vi "ConvertGoop1ToGoop3_KeepViPrefix.vi"(1 "OrgViName":path=path "C:/UML/GOOP2/AbstractNode_class/AbstractNode addChild.vi", 2 "ClassFolder":path=path "C:/UML/GOOP2/AbstractNode_class", 5 "error in (no error)":errorcluster, 6 "ClassPrefix":string="AbstractNode ") -> (12 "ClassFolderOut":path, 14 "Don'tUseVI":bool, 15 "KeepPrefix":bool, 16 "NewClassPath":path, 18 "NewClassPathWithPreFix":path, 19 "error out":errorcluster)   [LabVIEW 2020]
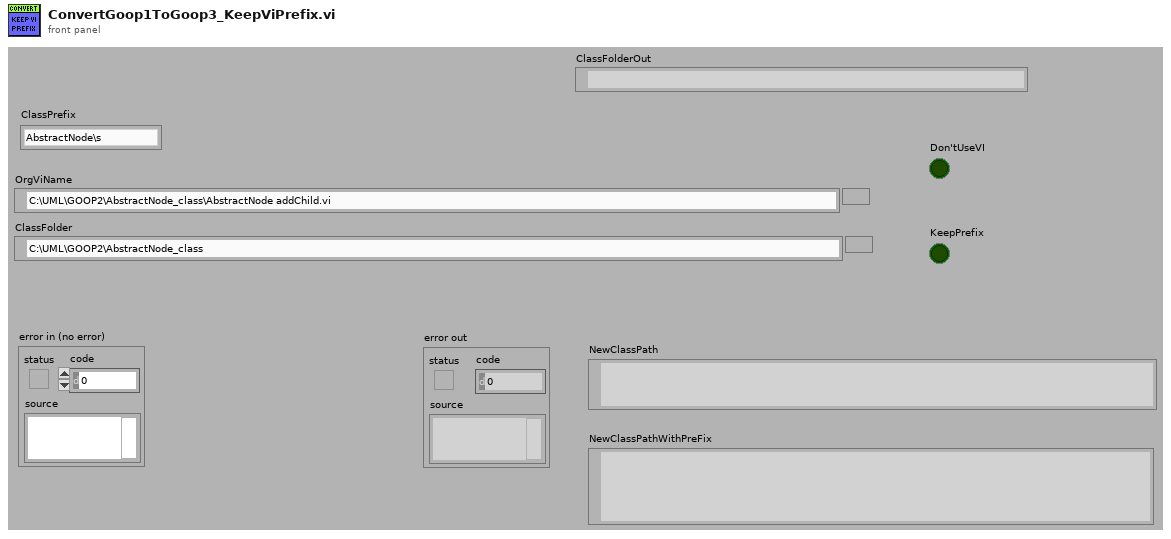
[diagram p1: front panel]
types:
  T1 = typedef "Librarian File Info Out.ctl" = cluster{"creation date":u32, "last mod date":u32, "type":string, "creator":string, "LV version":i32, "size":i32, "top level":bool}
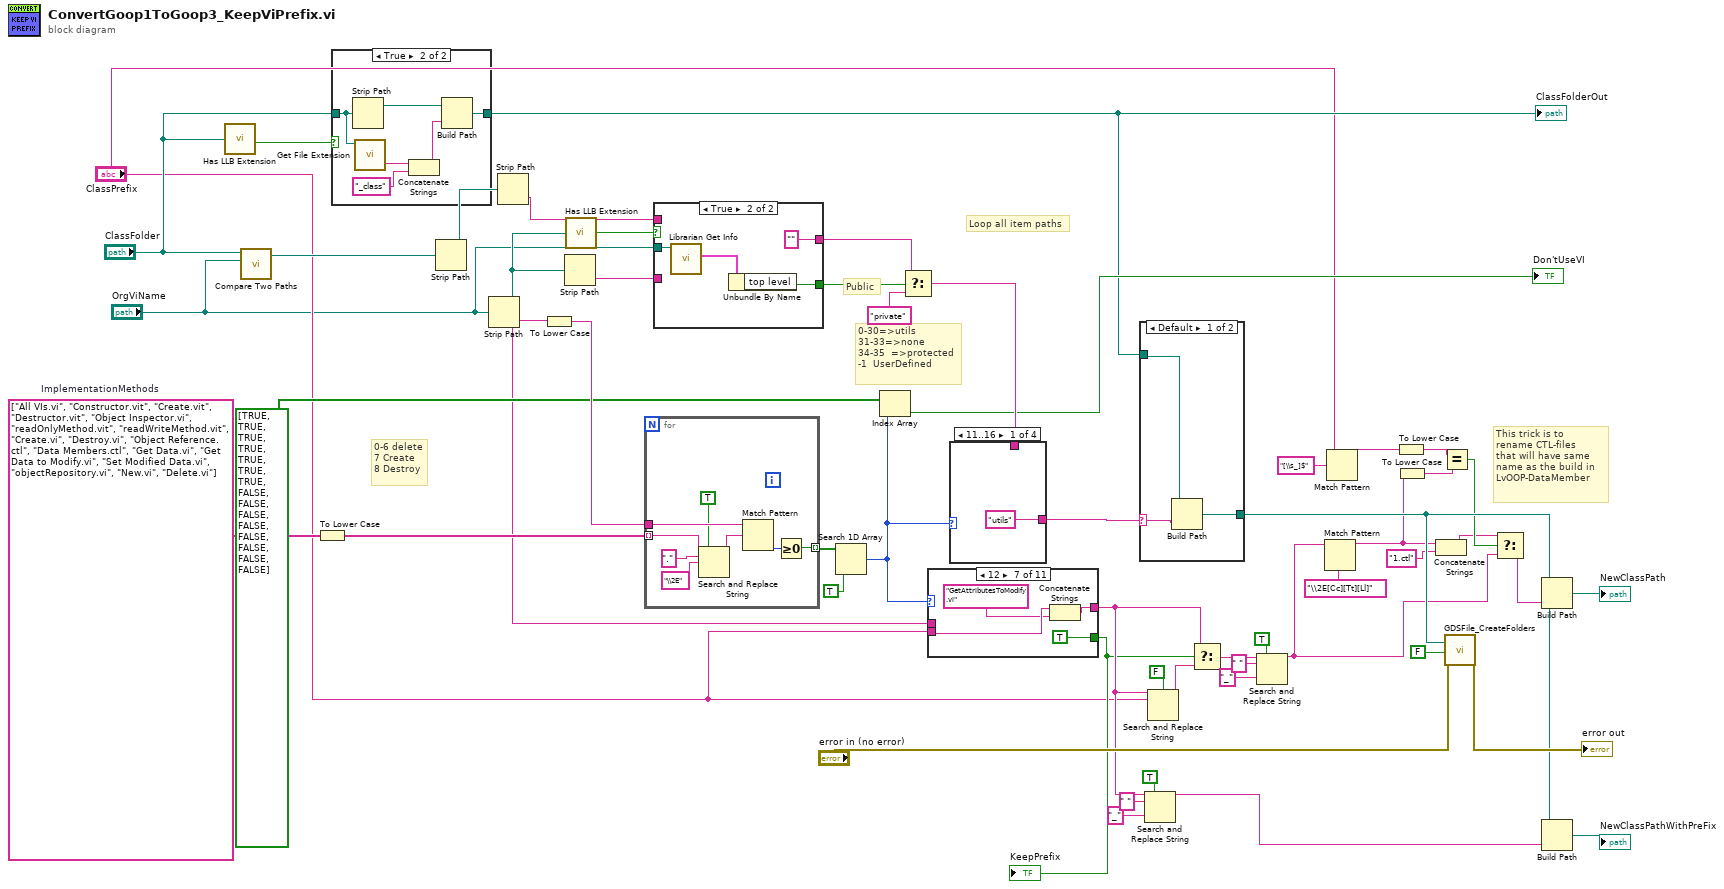
[diagram p0: block diagram]
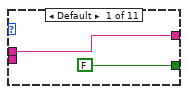
[diagram p2: hidden frame]
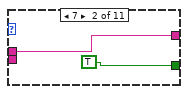
[diagram p3: hidden frame]
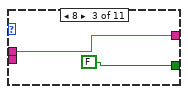
[diagram p4: hidden frame]
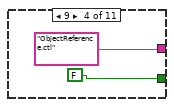
[diagram p5: hidden frame]
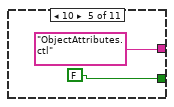
[diagram p6: hidden frame]
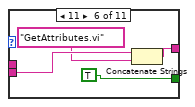
[diagram p7: hidden frame]
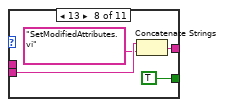
[diagram p8: hidden frame]
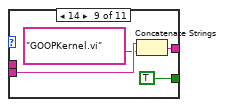
[diagram p9: hidden frame]
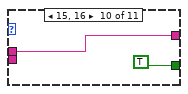
[diagram p10: hidden frame]
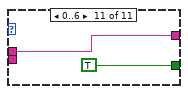
[diagram p11: hidden frame]
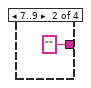
[diagram p14: hidden frame]
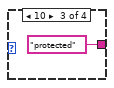
[diagram p15: hidden frame]
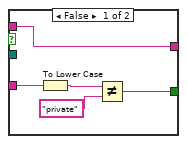
[diagram p17: hidden frame]
diagram:
  w53 = string[] ["All VIs.vi", "Constructor.vit", "Create.vit", "Destructor.vit", "Object Inspector.vi", "readOnlyMethod.vit", "readWriteMethod.vit", "Create.vi", "Destroy.vi", "Object Reference.ctl", "Data Members.ctl", "Get Data.vi", "Get Data to Modify.vi", "Set Modified Data.vi", "objectRepository.vi", "New.vi", "Delete.vi"]  # ImplementationMethods
  # "0-6 delete\n7 Create\n8 Destroy"
  # "This trick is to\nrename CTL-files\nthat will have same\nname as the build in\nLvOOP-DataMember"
  # "Public"
  # "0-30=>utils\n31-33=>none\n34-35  =>protected\n-1  UserDefined"
  # "Loop all item paths"
  n1 = call <vilib>:"Has LLB Extension.vi"("path"="ClassFolder") -> ("path to VI library?"=w20:bool)
  n2 = call <vilib>:"Compare Two Paths.vi"("Path 2"="OrgViName", "Path 1"="ClassFolder") -> ("Relative Path from 1 to 2"=w25:path)  [unwired: 6 in, 3 out]
  n3 = To Lower Case(string=w53) -> (all lower case string=w54:string[])
  n4 = case shown="True" w20 {
    tunnel: "ClassFolder" -> [w55 w61]
    tunnel: [w55 w60] -> w18
    frame False {
    }
    frame True {
      n5 = Strip Path(path=w61) -> (stripped path=w57:path)  [unwired: 1 out]
      n6 = call <vilib>:"Get File Extension.vi"("file"=w61) -> ("filename without extension"=w59:string)  [unwired: 6 in, 4 out]
      n7 = Concatenate Strings(w59, "_class" ("string")) -> (w56:string)
      n8 = Build Path(base path=w57, name or relative path=w56) -> (appended path=w60:path)
    }
  }
  "ClassFolderOut" <- w18
  n9 = Strip Path(path=w25) -> (stripped path=w24:path)  [unwired: 1 out]
  n10 = Strip Path(path="OrgViName") -> (stripped path=w50:path, name=w5:string)
  n11 = Strip Path(path=w24) -> (name=w23:string)  [unwired: 1 out]
  n12 = To Lower Case(string=w5) -> (all lower case string=w52:string)
  n13 = Strip Path(path=w50) -> (name=w47:string)  [unwired: 1 out]
  n14 = call <vilib>:"Has LLB Extension.vi"("path"=w50) -> ("path to VI library?"=w51:bool)
  n15 = for {
    tunnel: w54 -> [w68] mode=indexing
    tunnel: w52 -> [w69]
    tunnel: [w62] -> w38 mode=indexing
    n16 = Search and Replace String(replace all?=TRUE ("replace all? (F)"), input string=w68, search string=".", replace string="\\2E" ("replace string (\"\")")) -> (result string=w67:string)  [unwired: 4 in, 3 out]
    n17 = Match Pattern(string=w69, regular expression=w67) -> (offset past match=w63:i32)  [unwired: 1 in, 3 out]
    n18 = Greater Or Equal To 0?(x=w63) -> (x >= 0?=w62:bool)
  }
  n19 = case shown="True" w51 {
    tunnel: "OrgViName" -> [_ w78]
    tunnel: w47 -> [w70 _]
    tunnel: [w72 w76] -> w46
    tunnel: [w71 "" ("y")] -> w26
    tunnel: w23 -> [w71 _]
    frame False {
      n20 = To Lower Case(string=w70) -> (all lower case string=w74:string)
      n21 = Not Equal?(x=w74, y="private") -> (x != y?=w72:bool)
    }
    frame True {
      n22 = call <vilib>:"Librarian Get Info.vi"("path"=w78) -> ("file information"=w77:T1)  [unwired: 8 in, 2 out]
      n23 = Unbundle By Name(w77) -> ("top level"=w76:bool)
    }
  }
  n24 = Search 1D Array(1D array=w38, element=TRUE) -> (index of element=w6:i32)  [unwired: 1 in]
  n25 = Index Array(array=bool[] [TRUE, TRUE, TRUE, TRUE, TRUE, TRUE, TRUE, FALSE, FALSE, FALSE, FALSE, FALSE, FALSE, FALSE, FALSE] (".not. x?"), index=w6) -> (element=→"Don'tUseVI":bool)
  n26 = Select(t=w26, s=w46, f="private" ("y")) -> (s? t:f=w44:string)
  n27 = case shown="12" w6 {
    tunnel: w5 -> [w80 w82 w84 _ _ _ _ _ _ w106 w108]
    tunnel: [w80 w82 w84 "ObjectReference.ctl" ("name") "ObjectAttributes.ctl" ("name") w89 w93 w97 w101 w106 w108] -> w4
    tunnel: [FALSE ("replace all? (F)") TRUE ("ignore case? (F)") FALSE ("ignore case? (F)") FALSE ("ignore case? (F)") FALSE ("ignore case? (F)") TRUE ("ignore case? (F)") TRUE ("ignore case? (F)") TRUE ("ignore case? (F)") TRUE ("ignore case? (F)") TRUE ("ignore case? (F)") TRUE ("replace all? (F)")] -> w3
    tunnel: "ClassPrefix" -> [_ _ _ _ _ w91 w95 w99 w103 _ _]
    frame Default {
    }
    frame 7 {
    }
    frame 8 {
    }
    frame 9 {
    }
    frame 10 {
    }
    frame 11 {
      n28 = Concatenate Strings(w91, "GetAttributes.vi" ("name")) -> (w89:string)
    }
    frame 12 {
      n29 = Concatenate Strings(w95, "GetAttributesToModify.vi" ("name")) -> (w93:string)
    }
    frame 13 {
      n30 = Concatenate Strings(w99, "SetModifiedAttributes.vi" ("name")) -> (w97:string)
    }
    frame 14 {
      n31 = Concatenate Strings(w103, "GOOPKernel.vi" ("name")) -> (w101:string)
    }
    frame 15, 16 {
    }
    frame 0..6 {
    }
  }
  "KeepPrefix" <- w3
  n32 = case shown="11..16" w6 {
    tunnel: ["utils" "" "protected" w112] -> w43
    tunnel: w44 -> [_ _ _ w112]
    frame 11..16 {
    }
    frame 7..9 {
    }
    frame 10 {
    }
    frame Default {
    }
  }
  n33 = case shown="Default" w43 {
    selector: w43 -> [w114 _]
    tunnel: w18 -> [w115 w116]
    tunnel: [w113 w116] -> w33
    frame Default {
      n34 = Build Path(base path=w115, name or relative path=w114) -> (appended path=w113:path)
    }
    frame "" {
    }
  }
  n35 = Search and Replace String(replace all?=TRUE ("replace all? (F)"), input string=w4, search string=" ", replace string="_" ("replace string (\"\")")) -> (result string=w28:string)  [unwired: 4 in, 3 out]
  n36 = Search and Replace String(case sensitive?=FALSE ("ignore case? (F)"), input string=w4, search string="ClassPrefix") -> (result string=w49:string)  [unwired: 5 in, 3 out]
  n37 = Select(t=w4, s=w3, f=w49) -> (s? t:f=w29:string)
  n38 = Search and Replace String(replace all?=TRUE ("replace all? (F)"), input string=w29, search string=" ", replace string="_" ("replace string (\"\")")) -> (result string=w8:string)  [unwired: 4 in, 3 out]
  n39 = Match Pattern(string=w8, regular expression="\\2E[Cc][Tt][Ll]") -> (before substring=w11:string)  [unwired: 1 in, 3 out]
  n40 = Match Pattern(string="ClassPrefix", regular expression="[\\s_]$") -> (before substring=w16:string)  [unwired: 1 in, 3 out]
  n41 = To Lower Case(string=w16) -> (all lower case string=w14:string)
  n42 = To Lower Case(string=w11) -> (all lower case string=w15:string)
  n43 = Concatenate Strings(w11, "1.ctl" ("string")) -> (w9:string)
  n44 = Equal?(x=w14, y=w15) -> (x = y?=w12:bool)
  n45 = call "GDSFile_CreateFolders.vi"("Path"=w33, "Promt if folder\ndoes not exists?"=FALSE ("Promt if folder\ndoes not exists?"), "error in (no error)"="error in (no error)") -> ("error out"=→"error out":errorcluster)  [unwired: 12 in, 4 out]
  n46 = Select(t=w9, s=w12, f=w8) -> (s? t:f=w7:string)
  n47 = Build Path(base path=w33, name or relative path=w7) -> (appended path=→"NewClassPath":path)
  n48 = Build Path(base path=w33, name or relative path=w28) -> (appended path=→"NewClassPathWithPreFix":path)
